vi "test_button.vi"() -> ()   [LabVIEW 2020]
panel:
  in  "Boolean 2":bool
  in  "Boolean":bool
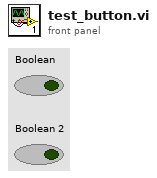
[diagram p1: front panel]
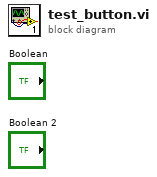
[diagram p0: block diagram]
diagram:
